vi "Cal Inst - Initialize.vi"(6 "Tab Control":T1(tab), 8 "error in (no error)":errorcluster, 9 "Voltage Level (0V)":dbl=120.0, 10 "Serial Configuration":cluster{"Baud Rate":u32, "Flow Control":u16}={"Baud Rate"=460800, "Flow Control"=0} {"Flow Control" items=["None", "XON/XOFF", "RTS/CTS", "XON/XOFF & RTS/CTS", "DTR/DSR", "XON/XOFF & DTR/DSR"]; "Baud Rate" items=["9600"=9600, "19200"=19200, "38400"=38400, "57600"=57600, "115200"=115200, "230400"=230400, "460800"=460800]}, 11 "VISA Refnum in":refnum<visa-resource-name>) -> (0 "error out":errorcluster, 3 "VISA Refnum out":refnum<visa-resource-name>)   [LabVIEW 2013]
uses:
  Libraries/California Instruments iX Series/California Instruments iX Series.lvlib
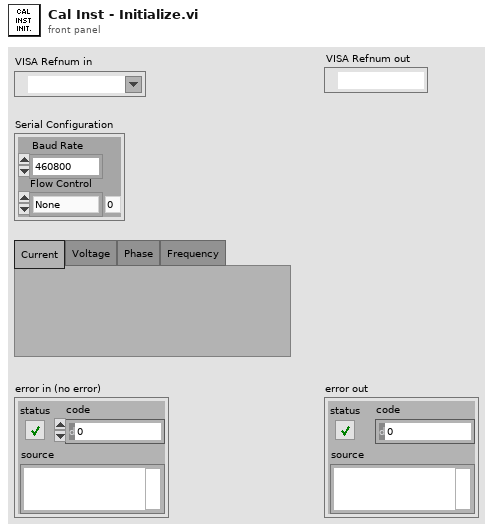
[diagram p1: front panel]
types:
  T1 = enum32{"Current", "Voltage", "Phase", "Frequency"}
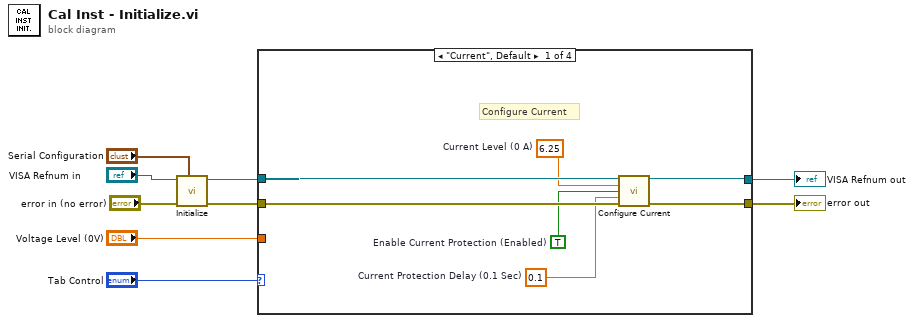
[diagram p0: block diagram]
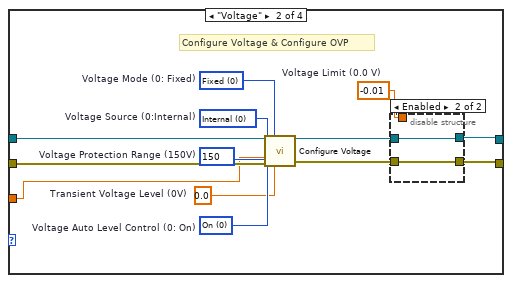
[diagram p2: hidden frame]
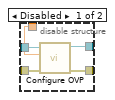
[diagram p3: hidden frame]
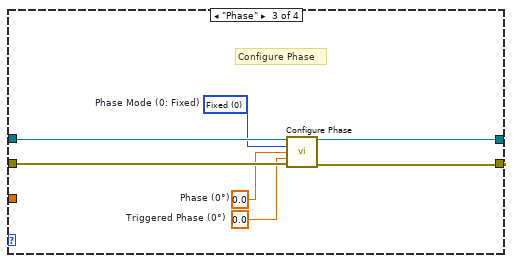
[diagram p4: hidden frame]
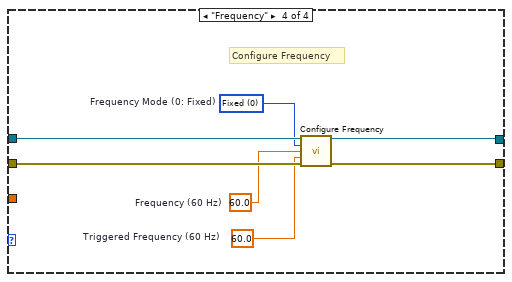
[diagram p5: hidden frame]
diagram:
  n1 = call "Initialize.vi"("Serial Configuration"="Serial Configuration", "error in (no error)"="error in (no error)", "VISA resource name"="VISA Refnum in") -> ("error out"=w5:errorcluster, "VISA resource name out"=w4:refnum<visa-resource-name>)  [unwired: 7 in]
  n2 = case shown="\"Current\", Default" "Tab Control" {
    tunnel: w4 -> [w16 w29 w43 w50]
    tunnel: w5 -> [w15 w28 w42 w49]
    tunnel: [w11 w19 w38 w45] -> w8
    tunnel: [w10 w18 w37 w44] -> w9
    tunnel: "Voltage Level (0V)" -> [_ w17 _ _]
    frame "Current", Default {
      w12 = 0.1  # Current Protection Delay (0.1 Sec)
      w13 = TRUE  # Enable Current Protection (Enabled)
      w14 = 6.25  # Current Level (0 A)
      # "Configure Current"
      n3 = call "Configure Current.vi"("VISA resource name"=w16, "Current Level (0 A)"=w14, "Enable Current Protection (Enabled)"=w13, "Current Protection Delay (0.1 Sec)"=w12, "error in (no error)"=w15) -> ("VISA resource name out"=w11:refnum<visa-resource-name>, "error out"=w10:errorcluster)  [unwired: 9 in]
    }
    frame "Voltage" {
      w20 = -0.01  # Voltage Limit (0.0 V)
      w23 = u16 150 items=["150"=150, "300"=300]  # Voltage Protection Range (150V)
      w26 = u16 0 items=["On", "Off", "Regulation"]  # Voltage Auto Level Control (0: On)
      w25 = u16 0 items=["Internal", "External"]  # Voltage Source (0:Internal)
      w27 = 0 items=["Fixed", "Step", "Pulse", "List"]  # Voltage Mode (0: Fixed)
      w24 = 0.0  # Transient Voltage Level (0V)
      # "Configure Voltage & Configure OVP"
      n4 = call "Configure Voltage.vi"("VISA resource name"=w29, "Voltage Mode (0: Fixed)"=w27, "Voltage Auto Level Control (0: On)"=w26, "Voltage Source (0:Internal)"=w25, "Voltage Level (0V)"=w17, "error in (no error)"=w28, "Transient Voltage Level (0V)"=w24, "Voltage Protection Range (150V)"=w23) -> ("VISA resource name out"=w22:refnum<visa-resource-name>, "error out"=w21:errorcluster)  [unwired: 6 in]
      n5 = disable-structure shown="Enabled" {
        disable-tunnel: w22 -> [w34 w36]
        disable-tunnel: w21 -> [w33 w35]
        disable-tunnel: w20 -> [w32 _]
        disable-tunnel: [w31 w36] -> w19
        disable-tunnel: [w30 w35] -> w18
        frame Disabled {
          n6 = call "Configure OVP.vi"("error in (no error)"=w33, "Voltage Limit (0.0 V)"=w32, "VISA resource name"=w34) -> ("error out"=w30:errorcluster, "VISA resource name out"=w31:refnum<visa-resource-name>)  [unwired: 7 in]
        }
        frame Enabled {
        }
      }
    }
    frame "Phase" {
      w39 = 0.0  # Triggered Phase (0°)
      w40 = 0.0  # Phase (0°)
      w41 = 0 items=["Fixed", "Step", "Pulse", "List"]  # Phase Mode (0: Fixed)
      # "Configure Phase"
      n7 = call "Configure Phase.vi"("VISA resource name"=w43, "Phase Mode (0: Fixed)"=w41, "Phase (0°)"=w40, "Triggered Phase (0°)"=w39, "error in (no error)"=w42) -> ("VISA resource name out"=w38:refnum<visa-resource-name>, "error out"=w37:errorcluster)  [unwired: 9 in]
    }
    frame "Frequency" {
      w46 = 60.0  # Triggered Frequency (60 Hz)
      w47 = 60.0  # Frequency (60 Hz)
      w48 = 0 items=["Fixed", "Step", "Pulse", "List", "Sense", "External"]  # Frequency Mode (0: Fixed)
      # "Configure Frequency"
      n8 = call "Configure Frequency.vi"("VISA resource name"=w50, "Frequency Mode (0: Fixed)"=w48, "Frequency (60 Hz)"=w47, "Triggered Frequency (60 Hz)"=w46, "error in (no error)"=w49) -> ("VISA resource name out"=w45:refnum<visa-resource-name>, "error out"=w44:errorcluster)  [unwired: 9 in]
    }
  }
  "error out" <- w9
  "VISA Refnum out" <- w8
